vi "Review Result.vi"(0 "Vector 18GHz Path in":refnum<class "Vector 18GHz Path.lvclass">, 11 "error in (no error)":errorcluster) -> (4 "Vector 18GHz Path out":refnum<class "Vector 18GHz Path.lvclass">, 6 "Response":string, 15 "error out":errorcluster)   [LabVIEW 2023, in "RFFixtureCharact.RFPM.lvlib" / "Vector 18GHz Path.lvclass"]
uses:
  Vector 18GHz Path.lvclass
  C:/rfcal/AuxTools/STSRFFixtureCharactUtility/Source/Code Modules/Common/Base Classes/Path/Path.lvclass
  Public/Base Classes/Vector/Vector Abstract Path/Type Definitions/Vector Charact Result.ctl
  <vilib>/Utility/error.llb/Trim Whitespace One-Sided.vi
  Vector 18GHz Path.lvclass/Vector 18GHz Path.ctl
  Public/Base Classes/Vector/Vector Abstract Path/Vector Abstract Path.lvclass
  Common/RFCalAndFixtureCharact.Common.lvlib
  Public/RFFixtureCharact.Public.lvlib
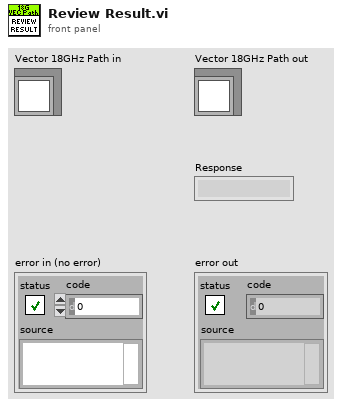
[diagram p1: front panel]
types:
  T1 = typedef "RFFixtureCharact.Public.lvlib/Vector Abstract Path.lvclass/Vector Charact Result.ctl" = cluster{"Port Power":dbl, "Frequency":dbl, "S Parameters":cdb[], "Out Of Limit":bool}
  T2 = typedef "RFFixtureCharact.RFPM.lvlib/Vector 18GHz Path Group.lvclass/Sweep.ctl" = cluster{"Port Power":dbl, "Frequencies":dbl[], "Reference Level":dbl, "IF Bandwidth":dbl}
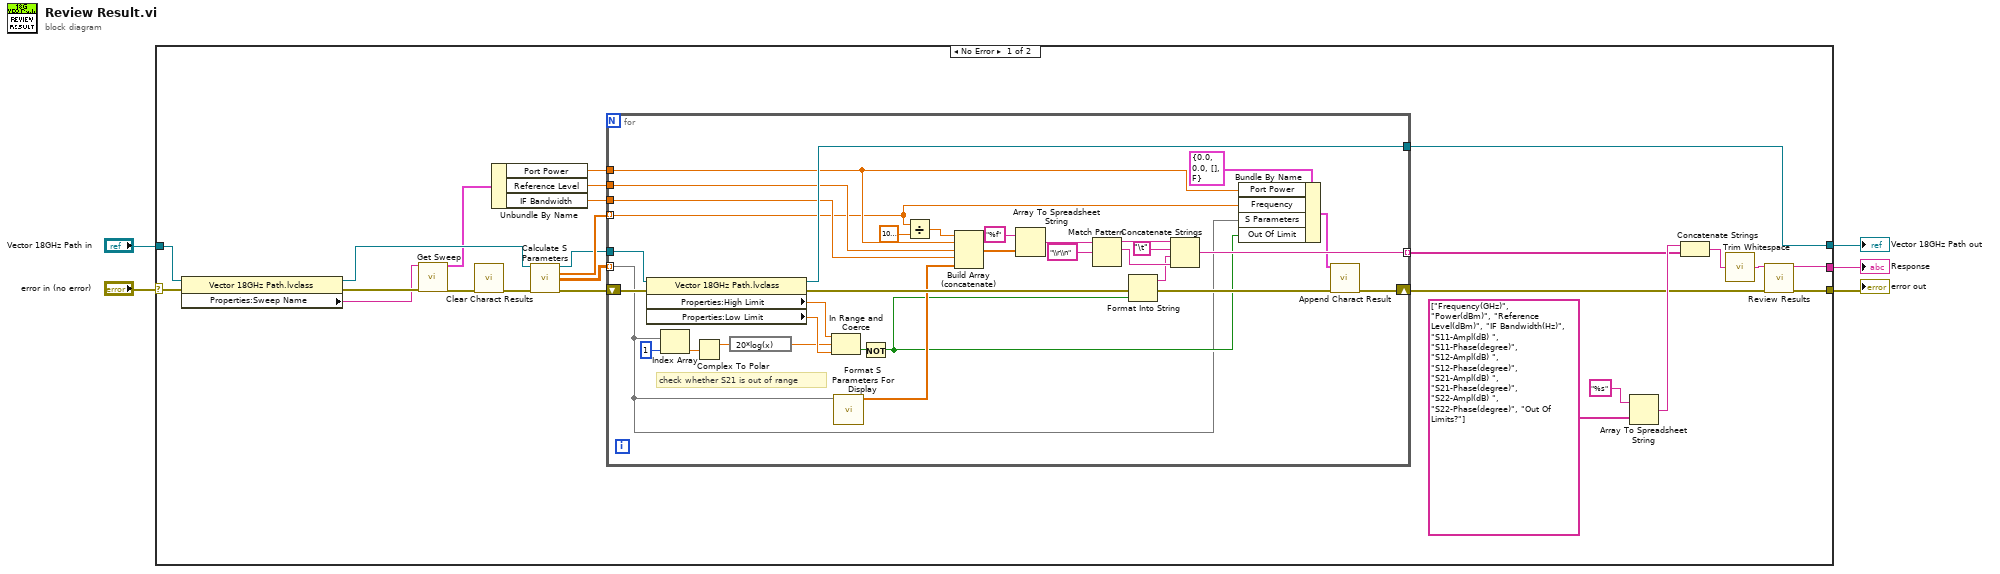
[diagram p0: block diagram]
diagram:
  n1 = case shown="No Error" "error in (no error)" {
    selector: "error in (no error)" -> [w26 w65]
    tunnel: [w23 w64] -> w2
    tunnel: [w24 _] -> w1
    tunnel: [w25 w65] -> w3
    tunnel: "Vector 18GHz Path in" -> [w30 w64]
    frame No Error {
      n2 = property class="Vector 18GHz Path.lvclass"(reference=w30, error in=w26) -> (reference out=w29:refnum<class "Vector 18GHz Path.lvclass">, error out=w28:errorcluster, "Properties:Sweep Name"=w27:string)
      n3 = call "Get Sweep.vi"("Sweep Name"=w27, "error in (no error)"=w28) -> ("Grid"=w22:T2, "error out"=w7:errorcluster)  [unwired: 11 in, 1 out]
      n4 = call "Clear Charact Results.vi"("error in"=w7) -> ("error out"=w6:errorcluster)  [unwired: 14 in]
      n5 = Unbundle By Name(w22) -> ("Port Power"=w20:dbl, "Reference Level"=w21:dbl, "IF Bandwidth"=w8:dbl)
      n6 = call-dynamic "Calculate S Parameters.vi"("Vector Path in"=w29, "error in (no error)"=w6) -> ("Vector Path out"=w10:refnum<class "Vector 18GHz Path.lvclass">, "Frequencies"=w19:dbl[], "S Parameters out"=w18:cdb[][], "error out"=w9:errorcluster)  [unwired: 10 in]
      n7 = for {
        shift-right: [w38] -> w12
        shift-left: w9 -> [w63]
        tunnel: w19 -> [w34] mode=indexing
        tunnel: w18 -> [w31] mode=indexing
        tunnel: w10 -> [w62]
        tunnel: w21 -> [w43]
        tunnel: w20 -> [w35]
        tunnel: [w54] -> w23
        tunnel: [w41] -> w11 mode=indexing
        tunnel: w8 -> [w40]
        # "check whether S21 is out of range"
        n8 = property class="Vector 18GHz Path.lvclass"(reference=w62, error in=w63) -> (reference out=w54:refnum<class "Vector 18GHz Path.lvclass">, error out=w42:errorcluster, "Properties:High Limit"=w58:dbl, "Properties:Low Limit"=w57:dbl)
        n9 = Index Array(array=w31, index=1) -> (element=w60:cdb)
        n10 = Complex To Polar(r * e^(i*theta)=w60) -> (r=w56:dbl)  [unwired: 1 out]
        n11 = expression code="20*log(x)"(w56) -> (w55:dbl)
        n12 = In Range and Coerce(upper limit=w58, x=w55, lower limit=w57) -> (In Range?=w59:bool)  [unwired: 1 out]
        n13 = call "Format S Parameters For Display.vi"("S Parameters"=w31) -> ("S Parameters For Display"=w33:dbl[])  [unwired: 14 in]
        n14 = Not(x=w59) -> (.not. x?=w32:bool)
        n15 = Divide(x=w34, y=1000000000.0) -> (x/y=w52:dbl)
        n16 = Build Array (concatenate)(w52, w35, w43, w40, w33) -> (w48:dbl[])
        n17 = Array To Spreadsheet String(array=w48, 3:"%f" ("format string")) -> (spreadsheet string=w50:string)  [unwired: 1 in]
        n18 = Match Pattern(string=w50, regular expression="\\r\\n") -> (before substring=w47:string, match substring=w45:string)  [unwired: 1 in, 2 out]
        n19 = Format Into String(error in=w42, w32) -> (resulting string=w44:string, error out=w39:errorcluster)  [unwired: 2 in]
        n20 = Concatenate Strings(w47, "\t", w44, w45) -> (w41:string)
        n21 = Bundle By Name(cluster=T1 {"Port Power"=0.0, "Frequency"=0.0, "S Parameters"=[], "Out Of Limit"=FALSE} ("Charact Result"), "Port Power"=w35, "Frequency"=w34, "S Parameters"=w31, "Out Of Limit"=w32) -> (w37:T1)
        n22 = call "Append Charact Result.vi"("Path cal resut in"=w37, "error in (no error)"=w39) -> ("error out"=w38:errorcluster)  [unwired: 13 in]
      }
      n23 = Array To Spreadsheet String(array=string[] ["Frequency(GHz)", "Power(dBm)", "Reference Level(dBm)", "IF Bandwidth(Hz)", "S11-Ampl(dB) ", "S11-Phase(degree)", "S12-Ampl(dB) ", "S12-Phase(degree)", "S21-Ampl(dB) ", "S21-Phase(degree)", "S22-Ampl(dB) ", "S22-Phase(degree)", "Out Of Limits?"], 3:"%s" ("format string")) -> (spreadsheet string=w15:string)  [unwired: 1 in]
      n24 = Concatenate Strings(w15, w11) -> (w14:string)
      n25 = call <vilib>:"Trim Whitespace.vi"("string"=w14) -> ("trimmed string"=w13:string)  [unwired: 1 in]
      n26 = call "Review Results.vi"("Cal Results"=w13, "error in (no error)"=w12) -> ("Response"=w24:string, "error out"=w25:errorcluster)  [unwired: 12 in]
    }
    frame Error {
    }
  }
  "error out" <- w3
  "Vector 18GHz Path out" <- w2
  "Response" <- w1
